vi "Read ROB info cluster element.vi"(8 "error in (no error)":errorcluster, 10 "Channel":i32, 11 "ROB info clusters":T3) -> (0 "error out":errorcluster, 1 "ROB infocluster ref":T1, 2 "ROB Info-display":T2={"ID:"=-1, "State:"="UNKNOWN", "Voltages"=0, "Temp:"=-1.0, "Latch count:"=-1, "VRef:"=enum."Unknown", "Trigthres:"=0, "MPPC EN"=FALSE, "Test charge"=FALSE, "Responding"=FALSE, "Last update"=timestamp(0 s since 1904-01-01)} {"Last update" format="%<%X>T"; "Trigthres:" format="%.0fmV"; "Temp:" format="%.2f C"}, 3 "ROB info clusters":T3)   [LabVIEW 2016]
uses:
  Typedefs/All ROBs info cluster refnum.ctl
  Typedefs/ROB display info.ctl
  Typedefs/ROB info refnum.ctl
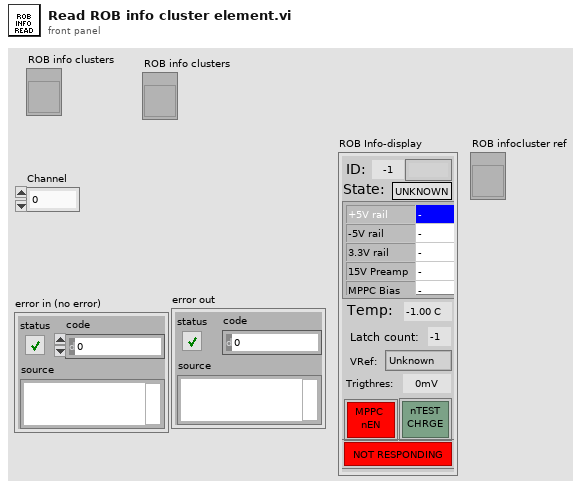
[diagram p1: front panel]
types:
  T1 = typedef "ROB info refnum.ctl" = refnum<vi>
  T2 = typedef "ROB display info.ctl" = cluster{"ID:":i32, "State:":string, "Voltages":i32, "Temp:":dbl, "Latch count:":i32, "VRef:":enum16{"External", "Internal", "Unknown"}, "Trigthres:":i32, "MPPC EN":bool, "Test charge":bool, "Responding":bool, "Last update":timestamp}
  T3 = typedef "All ROBs info cluster refnum.ctl" = refnum<vi>
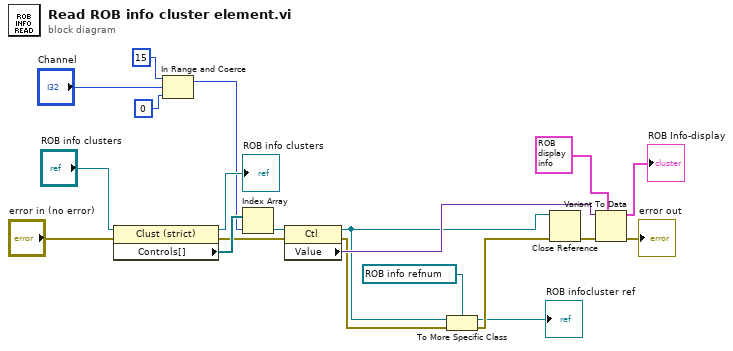
[diagram p0: block diagram]
diagram:
  n1 = property class="Clust (strict)"(reference="ROB info clusters", error in="error in (no error)") -> (reference out=→"ROB info clusters":T3, error out=w15:errorcluster, "Controls[]"=w19:refnum<vi>[])
  n2 = In Range and Coerce(upper limit=i8 15, x="Channel", lower limit=i8 0 ("upper limit")) -> (coerced(x)=w3:i32)  [unwired: 1 out]
  n3 = Index Array(array=w19, index=w3) -> (element=w18:refnum<vi>)
  n4 = property class="Ctl"(reference=w18, error in=w15) -> (reference out=w8:refnum<vi>, error out=w7:errorcluster, "Value"=w17:variant)
  n5 = To More Specific Class(target class=T1 refnum ("ROB infocluster ref"), reference=w8, error in=w7) -> (specific class reference=→"ROB infocluster ref":T1, error out=w6:errorcluster)
  n6 = Close Reference(reference=w8, error in (no error)=w6) -> (error out=w12:errorcluster)
  n7 = Variant To Data(error in=w12, type=T2 {"ID:"=0, "State:"="", "Voltages"=0, "Temp:"=0.0, "Latch count:"=0, "VRef:"=enum."External", "Trigthres:"=0, "MPPC EN"=FALSE, "Test charge"=FALSE, "Responding"=FALSE, "Last update"=timestamp(0 s since 1904-01-01)} ("ROB Info-display"), Variant=w17) -> (data=→"ROB Info-display":T2, error out=→"error out":errorcluster)
